vi "DCMotorBrakingStrengthChangeEventClose.vi"(8 "error in (no error)":errorcluster, 10 "Event Registration Refnum In":refnum<event-registration>, 11 "Devices In":u64[](array[numeric])) -> (0 "error out":errorcluster, 3 "Devices Out":u64[](array[numeric]))   [LabVIEW 2012, in "Phidget DC Motor.lvlib"]
doc: "${BrakingStrengthChange:CloseHeader}"
uses:
  <instrlib>/Phidgets/Phidget DC Motor/Phidget DC Motor.lvlib
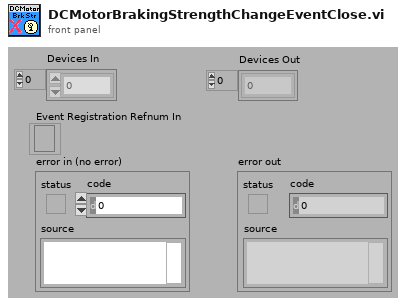
[diagram p1: front panel]
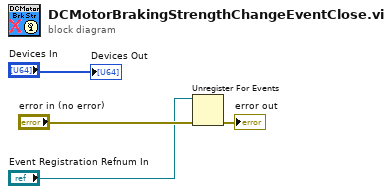
[diagram p0: block diagram]
diagram:
  n1 = Unregister For Events(event registration refnum="Event Registration Refnum In", error in="error in (no error)") -> (error out=→"error out":errorcluster)
  "Devices Out" <- "Devices In"
